vi "Load Becker-Hickl Data Headers.vi"(8 "Error In":errorcluster, 9 "# Data Blocks":i16 format="%.0x", 10 "Data Block Offset":i32, 11 "File Path Control":path) -> (0 "Error Out":errorcluster, 1 "Data Block Types":T1[](array[typedef]), 2 "Data Block Headers":T5[](array[typedef]) {"Block Type" format="%.0b"; "Long Block Number" format="%.0b"}, 3 "File Path":path, 4 "Compressed":bool[](array[boolean]))   [LabVIEW 2021, in "Becker-Hickl Files.lvlib"]
uses:
  Becker-Hickl Files.lvlib
  Becker-Hickl Data Block Header.ctl
  Becker-Hickl Data Block Type.ctl
  Becker-Hickl Data Creation Mode.ctl
  Becker-Hickl Data Block Content.ctl
  Becker-Hickl Data Type.ctl
  Becker-Hickl Read Single U16.vi
  Becker-Hickl Read Single U32.vi
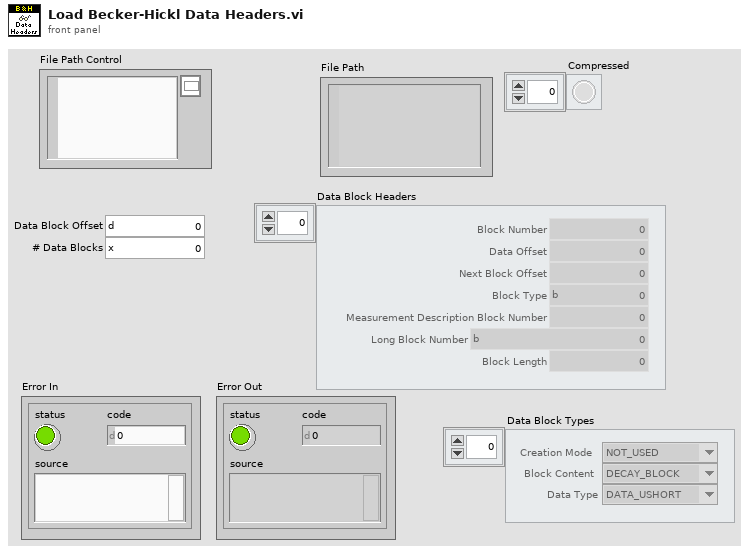
[diagram p1: front panel]
types:
  T1 = typedef "Becker-Hickl Files.lvlib/Becker-Hickl Data Block Type.ctl" = cluster{"Creation Mode":T2, "Block Content":T3, "Data Type":T4}
  T2 = typedef "Becker-Hickl Files.lvlib/Becker-Hickl Data Creation Mode.ctl" = enum16{"NOT_USED", "MEAS_DATA", "FLOW_DATA", "MEAS_DATA_FROM_FILE", "CALC_DATA", "SIM_DATA", "FIFO_DATA", "FIFO_DATA_FROM_FILE"}
  T3 = typedef "Becker-Hickl Files.lvlib/Becker-Hickl Data Block Content.ctl" = enum16{"DECAY_BLOCK", "PAGE_BLOCK", "FCS_BLOCK", "FIDA_BLOCK", "FILDA_BLOCK", "MCS_BLOCK", "IMG_BLOCK"}
  T4 = typedef "Becker-Hickl Files.lvlib/Becker-Hickl Data Type.ctl" = enum16{"DATA_USHORT", "DATA_ULONG", "DATA_DBL"}
  T5 = typedef "Becker-Hickl Files.lvlib/Becker-Hickl Data Block Header.ctl" = cluster{"Block Number":u16, "Data Offset":u32, "Next Block Offset":u32, "Block Type":u16, "Measurement Description Block Number":u16, "Long Block Number":u32, "Block Length":u32}
  T6 = enum16{"block_no", "data_offs", "next_block_offs", "block_type", "meas_desc_block_no", "lblock_no", "block_length"}
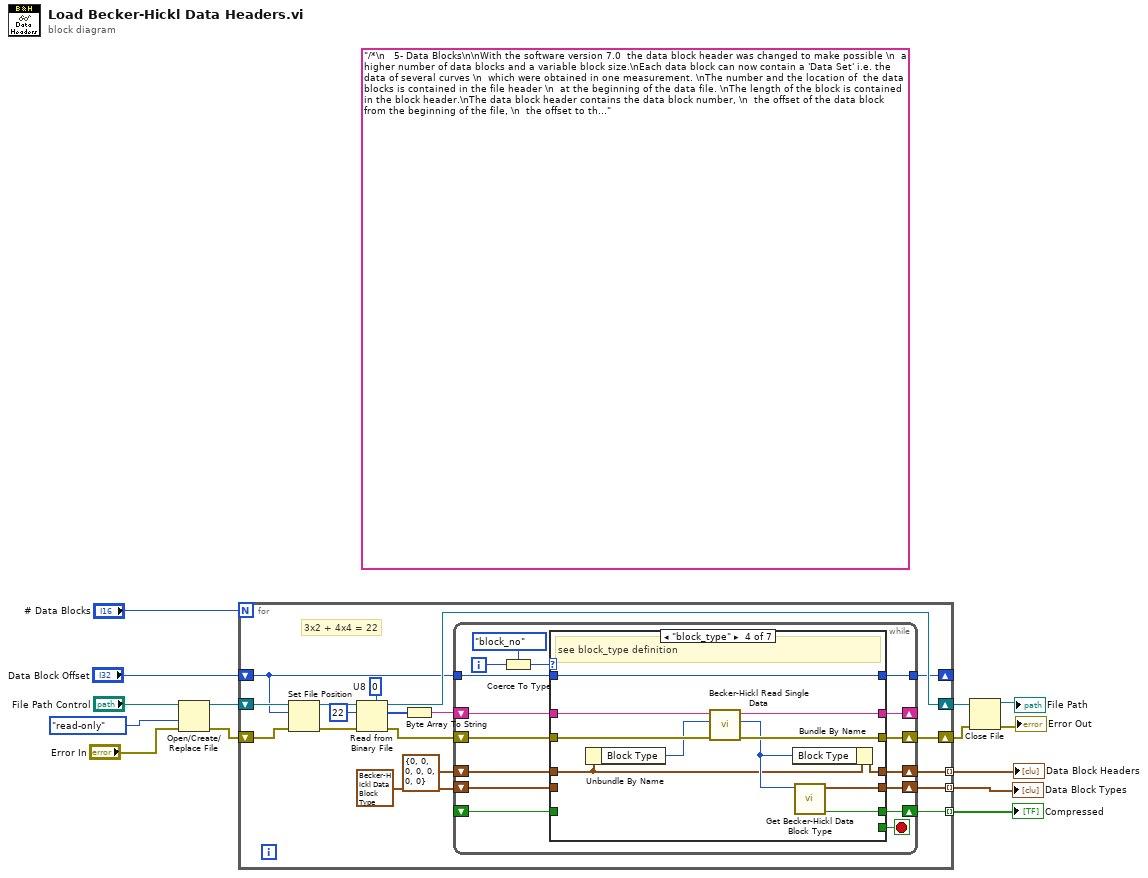
[diagram p0: block diagram]
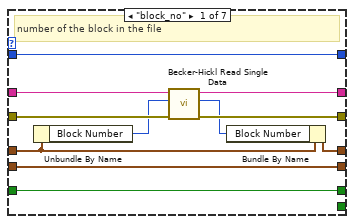
[diagram p2: hidden frame]
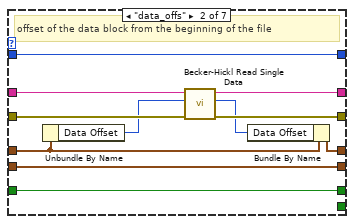
[diagram p3: hidden frame]
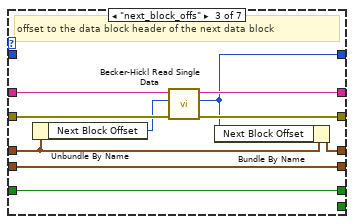
[diagram p4: hidden frame]
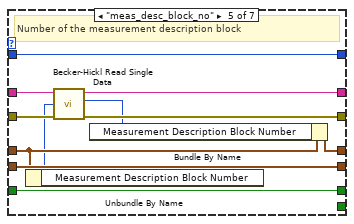
[diagram p5: hidden frame]
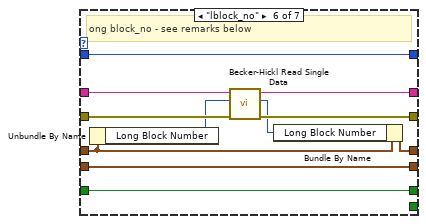
[diagram p6: hidden frame]
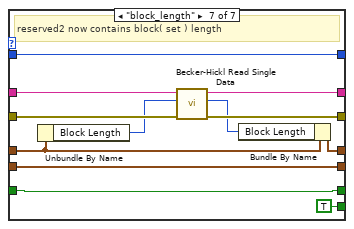
[diagram p7: hidden frame]
diagram:
  (unwired) "/*\n   5- Data Blocks\n\nWith the software version 7.0  the data block header was changed to make possible \n  a higher number of data blocks and a variable block size.\nEach data block can now contain a 'Data Set' i.e. the data of several curves \n  which were obtained in one measurement. \nThe number and the location of  the data blocks is contained in the file header \n  at the beginning of the data file. \nThe length of the block is contained in the block header.\nThe data block header contains the data block number, \n  the offset of the data block from the beginning of the file, \n  the offset to the next data block, \n  an information about the data in the block (measured block, block loaded from file, etc.), \n  and a reference to the corresponding measurement description block\n\nThe data block header structure is shown below.\n*/\n\n\ntypedef struct {\n   short          block_no;   // number of the block in the file\n                         // valid only  when in 0 .. 0x7ffe range, otherwise use lblock_no field\n                         // obsolete now, lblock_no contains full block no information                         \n   long           data_offs;       // offset of the data block from the beginning of the file\n   long           next_block_offs; // offset to the data block header of the next data block\n   unsigned short block_type;      // see block_type defines below\n   short          meas_desc_block_no; // Number of the measurement description block \n                                      //    corresponding to this data block\n   unsigned long  lblock_no;       // long block_no - see remarks below \n   unsigned long  block_length;    // reserved2 now contains block( set ) length\n   }BHFileBlockHeader;\n\n//    ( MSB bit is 31, LSB bit is 0 )\n//    The field block_no is obsolete\n//    The field 'lblock_no' contains the data block / data set number in the bits 0 to 23 \n//          and the module number (0 to 3) in the bits 24 to 25.\n//\n//    Block numbering start always from 1, so before calculating position in SPC memory \n//         ( or extracting FCS auto/cross rout. channels ) it should be at first decremented by 1\n//    \n//    for data set ( PAGE_BLOCK ) \n//           bits 0 - 23 represent number of the 1st block (decay curve) of the page\n//\n//    for FIFO_DATA \n//         bits 23 - 20   = block contents - the same as bits 4-7 in block_type\n//                          ( starting from software version 8.3 )\n//         for FIDA_BLOCK , FILDA_BLOCK, MCS_BLOCK and IMG_BLOCK\n//             bits 7 - 0  represent routing channel number\n//         for FCS_BLOCK bits 17 - 0  contain routing channel and module \n//                                      for auto and cross FCS\n//             bits 17 - 16   = Cross FCS module number\n//             bits 15 - 8    = rout. channel number   \n//             bits  7 - 0    = Cross FCS rout. channel number   \n//             when chan = cross_chan and mod == cross_mod - Auto FCS, \n//                           otherwise - Cross FCS\n\n\n//////////\n// defines for block type field in BHFileBlockHeader\n/////////\n\n// bits 0 - 3  in block_type define mode of creation\n\n#define NOT_USED              0\n#define MEAS_DATA             1   // normal measurement modes\n#define FLOW_DATA             2   // continuos flow measurement ( BIFL )  \n#define MEAS_DATA_FROM_FILE   3\n#define CALC_DATA             4   // calculated data\n#define SIM_DATA              5   // simulated data\n#define FIFO_DATA             8   // FIFO mode data\n#define FIFO_DATA_FROM_FILE   9   // FIFO mode data\n\n// bits 4 - 7  in block_type define block contents \n\n#define DECAY_BLOCK    0x0     // one decay curve\n#define PAGE_BLOCK     0x10    // set of decay curves = measured page\n#define FCS_BLOCK      0x20    // FCS histogram curve                 \n#define FIDA_BLOCK     0x30    // FIDA histogram curve                 \n#define FILDA_BLOCK    0x40    // FILDA histogram curve                 \n#define MCS_BLOCK      0x50    // MCS histogram curve                 \n#define IMG_BLOCK      0x60    // fifo image - set of curves          \n\n\n// bits 8 - 11 in block_type define data type      \n\n#define DATA_USHORT           0x0     // 16-bit unsigned short\n                                      //   (it was the only type up to 20.08.04)\n#define DATA_ULONG            0x100   // 32-bit unsigned long, for FIFO decay vcurves                                 \n#define DATA_DBL              0x200   // 32-bit double, for histogram data blocks \n\n// bits 12- 15 in block_type are not yet defined, reserved for future use\n         \n      // defines for page data sets\n#define MEAS_PAGE             0x11\n#define FLOW_PAGE             0x12\n#define MEAS_PAGE_FROM_FILE   0x13\n#define CALC_PAGE             0x14\n#define SIM_PAGE              0x15\n\n"
  n1 = Open/Create/Replace File(file path (use dialog)="File Path Control", error in="Error In", access (0:read/write)=enum16{"read/write", "read-only", "write-only"}."read-only") -> (refnum out=w11:refnum<file>, error out=w10:errorcluster)  [unwired: 3 in, 1 out]
  n2 = for {
    N: "# Data Blocks" -> [_]
    tunnel: [w23] -> w8 mode=indexing
    shift-right: [w24] -> w6
    shift-left: w10 -> [w28]
    shift-right: [w21] -> w7
    shift-left: w11 -> [w29]
    shift-right: [w20] -> _
    shift-left: "Data Block Offset" -> [w19]
    tunnel: [w18] -> w2 mode=indexing
    tunnel: [w15] -> w1 mode=indexing
    w32 = u8 0  # U8
    # "3x2 + 4x4 = 22"
    n3 = Set File Position(offset (in bytes) (0)=w19, refnum=w29, error in=w28) -> (refnum out=w27:refnum<file>, error out=w26:errorcluster)  [unwired: 1 in]
    n4 = Read from Binary File(5:w32, 8:w26, 10:22 ("count (1)"), 11:w27) -> (0:w22:errorcluster, 2:w30:u8[], 3:w21:refnum<file>)  [unwired: 2 in, 1 out]
    n5 = Byte Array To String(unsigned byte array=w30) -> (string=w16:string)
    n6 = while {
      shift-right: [w43] -> w24
      shift-left: w22 -> [w47]
      shift-right: [w42] -> _
      shift-left: w16 -> [w46]
      shift-right: [w44] -> w23
      shift-left: T5 {"Block Number"=0, "Data Offset"=0, "Next Block Offset"=0, "Block Type"=0, "Measurement Description Block Number"=0, "Long Block Number"=0, "Block Length"=0} ("Data Block Header") -> [w45]
      tunnel: [w41] -> w20
      tunnel: w19 -> [w40]
      shift-right: [w39] -> w18
      shift-left: T1 {"Creation Mode"=enum."NOT_USED", "Block Content"=enum."DECAY_BLOCK", "Data Type"=enum."DATA_USHORT"} ("Data Block Type") -> [w38]
      shift-right: [w34] -> w15
      shift-left: _ -> [w33]
      i -> [w48]
      stop <- w35 stop-if-true
      (unwired) FALSE
      (unwired) FALSE
      n7 = Coerce To Type(0:w48, 1:T6."block_no") -> (2:w37:T6)
      n8 = case shown="\"block_type\"" w37 {
        tunnel: w47 -> [w57 w68 w78 w89 w100 w111 w123]
        tunnel: w46 -> [w58 w69 w79 w90 w101 w112 w124]
        tunnel: w45 -> [w51 w62 w73 w83 w94 w105 w116]
        tunnel: [w59 w70 w80 w91 w102 w113 w125] -> w44
        tunnel: [w56 w67 w77 w88 w99 w110 w122] -> w43
        tunnel: [w55 w66 w76 w87 w98 w109 w121] -> w42
        tunnel: [w53 w64 w75 w86 w96 w107 w119] -> w41
        tunnel: w40 -> [w53 w64 _ w86 w96 w107 w119]
        tunnel: [w52 w63 w74 w84 w95 w106 w118] -> w39
        tunnel: w38 -> [w52 w63 w74 _ w95 w106 w118]
        tunnel: [_ _ _ _ _ _ TRUE] -> w35
        tunnel: [w49 w60 w71 w81 w92 w103 w114] -> w34
        tunnel: w33 -> [w49 w60 w71 _ w92 w103 w114]
        frame "block_no" {
          # "number of the block in the file"
          n9 = Unbundle By Name(w51) -> ("Block Number"=w50:u16)
          n10 = call-poly "Becker-Hickl Read Single Data.vi"("Error In"=w57, "Default"=w50, "Bytes in"=w58) -> ("Error Out"=w56:errorcluster, "U16"=w54:u16, "Bytes out"=w55:string)  [unwired: 6 in]
          n11 = Bundle By Name(cluster=w51, "Block Number"=w54) -> (w59:T5)
        }
        frame "data_offs" {
          # "offset of the data block from the beginning of the file"
          n12 = Unbundle By Name(w62) -> ("Data Offset"=w61:u32)
          n13 = call-poly "Becker-Hickl Read Single Data.vi"("Error In"=w68, "Default"=w61, "Bytes in"=w69) -> ("Error Out"=w67:errorcluster, "U32"=w65:u32, "Bytes out"=w66:string)  [unwired: 6 in]
          n14 = Bundle By Name(cluster=w62, "Data Offset"=w65) -> (w70:T5)
        }
        frame "next_block_offs" {
          # "offset to the data block header of the next data block"
          n15 = Unbundle By Name(w73) -> ("Next Block Offset"=w72:u32)
          n16 = call-poly "Becker-Hickl Read Single Data.vi"("Error In"=w78, "Default"=w72, "Bytes in"=w79) -> ("Error Out"=w77:errorcluster, "U32"=w75:u32, "Bytes out"=w76:string)  [unwired: 6 in]
          n17 = Bundle By Name(cluster=w73, "Next Block Offset"=w75) -> (w80:T5)
        }
        frame "block_type" {
          # "see block_type definition"
          n18 = Unbundle By Name(w83) -> ("Block Type"=w82:u16)
          n19 = call-poly "Becker-Hickl Read Single Data.vi"("Error In"=w89, "Default"=w82, "Bytes in"=w90) -> ("Error Out"=w88:errorcluster, "U16"=w85:u16, "Bytes out"=w87:string)  [unwired: 6 in]
          n20 = Bundle By Name(cluster=w83, "Block Type"=w85) -> (w91:T5)
          n21 = call "Get Becker-Hickl Data Block Type.vi"("Block Type"=w85) -> ("Compressed"=w81:bool, "Data Block Type"=w84:T1)  [unwired: 9 in]
        }
        frame "meas_desc_block_no" {
          # "Number of the measurement description block"
          n22 = Unbundle By Name(w94) -> ("Measurement Description Block Number"=w93:u16)
          n23 = call-poly "Becker-Hickl Read Single Data.vi"("Error In"=w100, "Default"=w93, "Bytes in"=w101) -> ("Error Out"=w99:errorcluster, "U16"=w97:u16, "Bytes out"=w98:string)  [unwired: 6 in]
          n24 = Bundle By Name(cluster=w94, "Measurement Description Block Number"=w97) -> (w102:T5)
        }
        frame "lblock_no" {
          # "ong block_no - see remarks below"
          n25 = Unbundle By Name(w105) -> ("Long Block Number"=w104:u32)
          n26 = call-poly "Becker-Hickl Read Single Data.vi"("Error In"=w111, "Default"=w104, "Bytes in"=w112) -> ("Error Out"=w110:errorcluster, "U32"=w108:u32, "Bytes out"=w109:string)  [unwired: 6 in]
          n27 = Bundle By Name(cluster=w105, "Long Block Number"=w108) -> (w113:T5)
        }
        frame "block_length" {
          # "reserved2 now contains block( set ) length"
          n28 = Unbundle By Name(w116) -> ("Block Length"=w115:u32)
          n29 = call-poly "Becker-Hickl Read Single Data.vi"("Error In"=w123, "Default"=w115, "Bytes in"=w124) -> ("Error Out"=w122:errorcluster, "U32"=w120:u32, "Bytes out"=w121:string)  [unwired: 6 in]
          n30 = Bundle By Name(cluster=w116, "Block Length"=w120) -> (w125:T5)
        }
      }
    }
  }
  "Data Block Headers" <- w8
  "Data Block Types" <- w2
  "Compressed" <- w1
  n31 = Close File(refnum=w7, error in=w6) -> (path=→"File Path":path, error out=→"Error Out":errorcluster)
